vi "PipBoy_NotifyBallonLabVIEWVersion.vi"(8 "error in (no error)":errorcluster, 10 "LabVIEWEventIn":T1, 11 "PipBoyDataIn":T3) -> (0 "error out":errorcluster, 2 "LabVIEWEventOut":T1, 3 "PipBoyDataOut":T3)   [LabVIEW 2014]
uses:
  ctls/PipBoy_PipBoyData.ctl
  ctls/PipBoy_ProcComm.ctl
  System.Windows.Forms
  ctls/PipBoy_PipBoyCommand.ctl
  ctls/PipBoy_Message.ctl
  modules/support/Message Queue/All Message Queues.ctl
  modules/support/Message Queue/Message Cluster.ctl
  ctls/PipBoy_FileConf.ctl
  ctls/PipBoy_PicComm.ctl
  ctls/PipBoy_GeneralParams.ctl
  ctls/PipBoy_Pages.ctl
  ctls/PipBoy_LabVIEWEvent.ctl
  ctls/PipBoy_DetectionType.ctl
  modules/support/Message Queue/Message Queue.lvlib
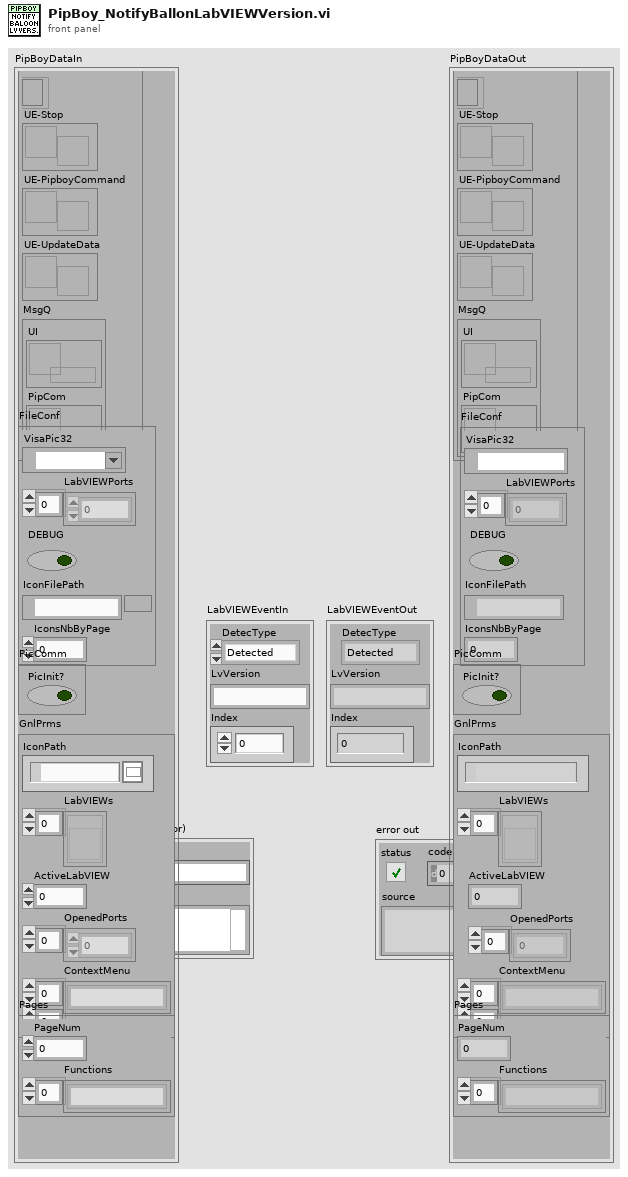
[diagram p1: front panel]
types:
  T1 = typedef "PipBoy_LabVIEWEvent.ctl" = cluster{"DetecType":T2, "LvVersion":string, "Index":i32}
  T2 = typedef "PipBoy_DetectionType.ctl" = enum16{"Detected", "Lost"}
  T3 = typedef "PipBoy_PipBoyData.ctl" = cluster{"ProcComm":T4, "FileConf":T6, "PicComm":T7, "GnlPrms":T8, "Pages":T9}
  T4 = typedef "PipBoy_ProcComm.ctl" = cluster{"NotifyIconRef":refnum<k24>, "UE-Stop":refnum<user-event>, "UE-PipboyCommand":refnum<user-event>, "UE-UpdateData":refnum<user-event>, "MsgQ":T5}
  T5 = typedef "Message Queue.lvlib/All Message Queues.ctl" = cluster{"UI":refnum<queue>, "PipCom":refnum<queue>}
  T6 = typedef "PipBoy_FileConf.ctl" = cluster{"VisaPic32":refnum<visa-resource-name>, "LabVIEWPorts":u16[], "DEBUG":bool, "IconFilePath":path, "IconsNbByPage":i32}
  T7 = typedef "PipBoy_PicComm.ctl" = cluster{"PicInit?":bool}
  T8 = typedef "PipBoy_GeneralParams.ctl" = cluster{"IconPath":path, "LabVIEWs":refnum<vi>[], "ActiveLabVIEW":i32, "OpenedPorts":u16[], "ContextMenu":string[][]}
  T9 = typedef "PipBoy_Pages.ctl" = cluster{"PageNum":i32, "Functions":string[]}
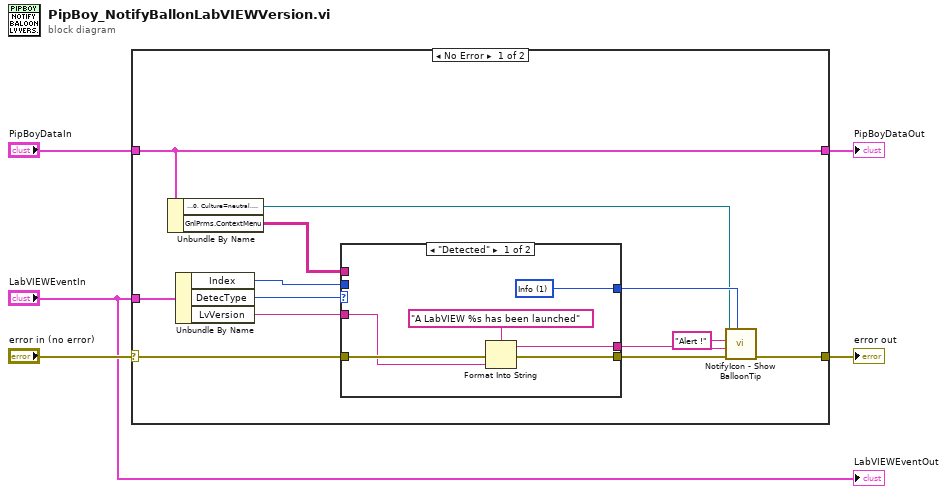
[diagram p0: block diagram]
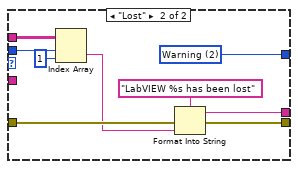
[diagram p2: hidden frame]
diagram:
  n1 = case shown="No Error" "error in (no error)" {
    selector: "error in (no error)" -> [w16 w35]
    tunnel: [w17 w35] -> w4
    tunnel: [w18 w34] -> w2
    tunnel: "PipBoyDataIn" -> [w18 w34]
    tunnel: "LabVIEWEventIn" -> [w15 _]
    frame No Error {
      n2 = Unbundle By Name(w18) -> ("ProcComm.NotifyIconRef"=w8:refnum<k24>, "GnlPrms.ContextMenu"=w7:string[][])
      n3 = Unbundle By Name(w15) -> ("Index"=w6:i32, "DetecType"=w10:T2, "LvVersion"=w14:string)
      n4 = case shown="\"Detected\"" w10 {
        tunnel: w16 -> [w24 w29]
        tunnel: w14 -> [w23 _]
        tunnel: [w21 w26] -> w12
        tunnel: [w20 w28] -> w11
        tunnel: [w19 w33] -> w9
        tunnel: w7 -> [_ w32]
        tunnel: w6 -> [_ w31]
        frame "Detected" {
          w19 = 1 items=["None", "Info", "Warning", "Error"] ("Icon (None) 2")
          n5 = Format Into String(format string="A LabVIEW %s has been launched" ("Title"), error in=w24, w23) -> (resulting string=w21:string, error out=w20:errorcluster)  [unwired: 1 in]
        }
        frame "Lost" {
          w33 = 2 items=["None", "Info", "Warning", "Error"] ("Icon (None) 2")
          n6 = Index Array(array=w32, index (row)=w31, index (col)=1 ("disabled index (col)")) -> (element=w25:string)
          n7 = Format Into String(format string="LabVIEW %s has been lost" ("Title"), error in=w29, w25) -> (resulting string=w26:string, error out=w28:errorcluster)  [unwired: 1 in]
        }
      }
      n8 = call <userlib>:"NotifyIcon - Show BalloonTip.vi"("Icon (None)"=w9, "error in"=w11, "Text"=w12, "Title"="Alert !", "NotifyIcon reference in"=w8) -> ("error out"=w17:errorcluster)  [unwired: 5 in, 1 out]
    }
    frame Error {
    }
  }
  "error out" <- w4
  "PipBoyDataOut" <- w2
  "LabVIEWEventOut" <- "LabVIEWEventIn"
